vi "niDTS WLAN INSTR TX Configure Basic.vi"(8 "error in (no error)":errorcluster, 10 "Channel Secondary Factor":enum16{"-1", "1", "0"}(ring)=enum."1", 11 "niDTS WLAN INSTR TX in":refnum<class "niDTS WLAN INSTR TX.lvclass">) -> (0 "error out":errorcluster, 3 "niDTS WLAN INSTR TX out":refnum<class "niDTS WLAN INSTR TX.lvclass">)   [LabVIEW 2015, in "niDTS WLAN.lvlib" / "niDTS WLAN INSTR TX.lvclass"]
doc: "Sets:\n\n* WlanStandard\n* ChannelBandwidth\n* MaxInputPower\n* CarrierFrequency"
uses:
  niDTS WLAN INSTR TX.lvclass
  niDTS WLAN INSTR TX.lvclass/niDTS WLAN INSTR TX.ctl
  RiviInstDriver/niRfsaWlan/Objects/niRfsaWlan.lvclass
  niDTS WLAN.lvlib
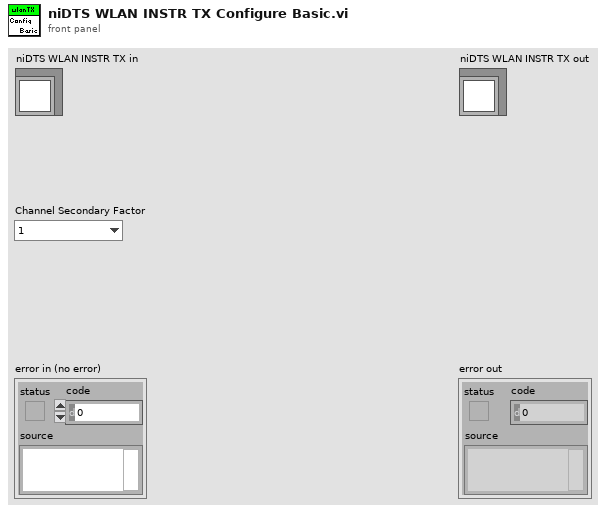
[diagram p1: front panel]
types:
  T1 = typedef "niRfsaWlan.lvclass/niRfsaWlan INC Handle.ctl" = refnum<data-value>
  T2 = typedef "niDTS WLAN.lvlib/niDTS WLAN INC Standard.ctl" = enum16{"802.11 b DSSS", "802.11 a/g OFDM", "802.11 n HT", "802.11 ac VHT"}
  T3 = typedef "niDTS WLAN.lvlib/niDTS WLAN INC CH BW.ctl" = enum16{"20 MHz", "40 MHz", "80 MHz", "160 MHz"}
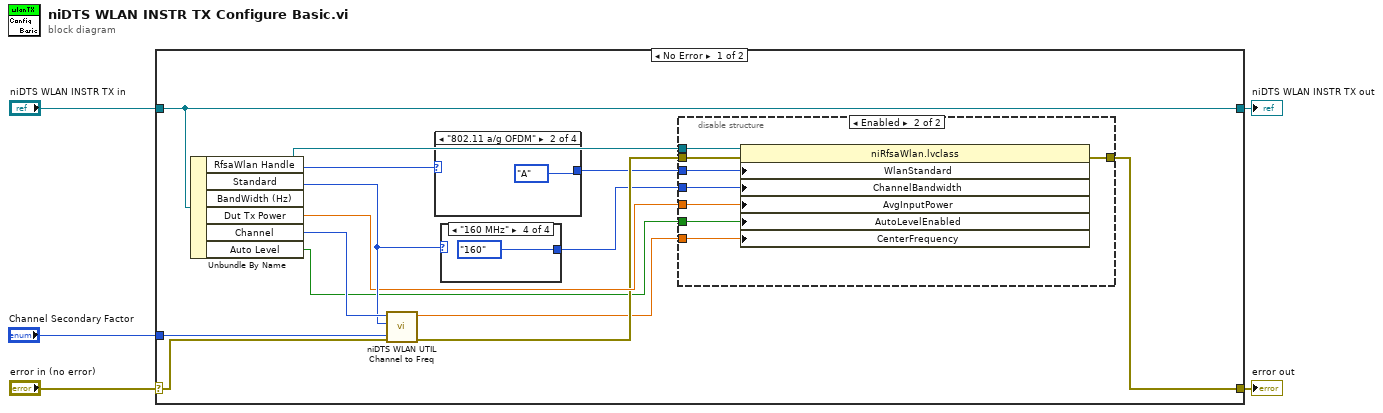
[diagram p0: block diagram]
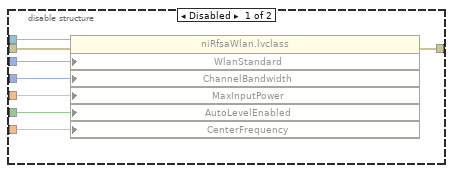
[diagram p2: hidden frame]
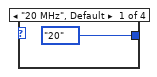
[diagram p3: hidden frame]
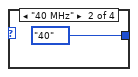
[diagram p4: hidden frame]
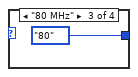
[diagram p5: hidden frame]
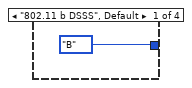
[diagram p6: hidden frame]
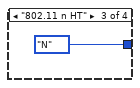
[diagram p7: hidden frame]
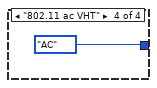
[diagram p8: hidden frame]
diagram:
  n1 = case shown="No Error" "error in (no error)" {
    selector: "error in (no error)" -> [w14 w45]
    tunnel: [w12 w45] -> w4
    tunnel: [w19 w44] -> w2
    tunnel: "niDTS WLAN INSTR TX in" -> [w19 w44]
    tunnel: "Channel Secondary Factor" -> [w13 _]
    frame No Error {
      n2 = Unbundle By Name(w19) -> ("RfsaWlan Handle"=w18:T1, "Standard"=w17:T2, "BandWidth (Hz)"=w15:T3, "Dut Tx Power"=w11:dbl, "Channel"=w16:i32, "Auto Level"=w7:bool)
      n3 = call "niDTS WLAN UTIL Channel to Freq.vi"("secondary factor"=w13, "error in"=w14, "CH BW"=w15, "Channel"=w16) -> ("error out"=w10:errorcluster, "Center Frequency (Hz)"=w6:dbl)  [unwired: 5 in, 1 out]
      n4 = case shown="\"802.11 a/g OFDM\"" w17 {
        tunnel: [enum16{"A", "B", "G", "N", "AC"}."B" ("CONFigure:RFSA:WLAN:WlanStandard") enum16{"A", "B", "G", "N", "AC"}."A" ("CONFigure:RFSA:WLAN:WlanStandard") enum16{"A", "B", "G", "N", "AC"}."N" ("CONFigure:RFSA:WLAN:WlanStandard") enum16{"A", "B", "G", "N", "AC"}."AC" ("CONFigure:RFSA:WLAN:WlanStandard")] -> w9
        frame "802.11 b DSSS", Default {
        }
        frame "802.11 a/g OFDM" {
        }
        frame "802.11 n HT" {
        }
        frame "802.11 ac VHT" {
        }
      }
      n5 = case shown="\"160 MHz\"" w15 {
        tunnel: [enum16{"5", "10", "20", "40", "80", "160"}."20" ("CONFigure:RFSA:WLAN:ChannelBandwidth") enum16{"5", "10", "20", "40", "80", "160"}."40" ("CONFigure:RFSA:WLAN:ChannelBandwidth") enum16{"5", "10", "20", "40", "80", "160"}."80" ("CONFigure:RFSA:WLAN:ChannelBandwidth") enum16{"5", "10", "20", "40", "80", "160"}."160" ("CONFigure:RFSA:WLAN:ChannelBandwidth")] -> w8
        frame "20 MHz", Default {
        }
        frame "40 MHz" {
        }
        frame "80 MHz" {
        }
        frame "160 MHz" {
        }
      }
      n6 = disable-structure shown="Enabled" {
        disable-tunnel: w18 -> [w27 w35]
        disable-tunnel: [w26 w34] -> w12
        disable-tunnel: w11 -> [w25 w33]
        disable-tunnel: w10 -> [w24 w32]
        disable-tunnel: w9 -> [w23 w31]
        disable-tunnel: w8 -> [w22 w30]
        disable-tunnel: w7 -> [w21 w29]
        disable-tunnel: w6 -> [w20 w28]
        frame Disabled {
          n7 = property class="niRfsaWlan.lvclass"(reference=w27, error in=w24, "WlanStandard"=w23, "ChannelBandwidth"=w22, "MaxInputPower"=w25, "AutoLevelEnabled"=w21, "CenterFrequency"=w20) -> (error out=w26:errorcluster)  [unwired: 1 out]
        }
        frame Enabled {
          n8 = property class="niRfsaWlan.lvclass"(reference=w35, error in=w32, "WlanStandard"=w31, "ChannelBandwidth"=w30, "AvgInputPower"=w33, "AutoLevelEnabled"=w29, "CenterFrequency"=w28) -> (error out=w34:errorcluster)  [unwired: 1 out]
        }
      }
    }
    frame Error {
    }
  }
  "error out" <- w4
  "niDTS WLAN INSTR TX out" <- w2
